vi "ModbusIRQTriggerLoop.vi"(11 "ModbusPortSettings":T1={"TxPort"="ModbusPort1Tx", "TxDataFIFO"="ModbusPort1TxFIFO", "TxInternalDataFIFO"="ModbusPort1TxInternalFIFO", "TxHealthAndStatusFIFO"="ModbusPort1TxHealthAndStatusFIFO", "RxPort"="ModbusPort1Rx", "RxDataFIFO"="ModbusPort1RxFIFO", "RxHealthAndStatusFIFO"="ModbusPort1RxHealthAndStatusFIFO", "WaitForRxFrameRegister"="ModbusPort1WaitForRxControl", "BaseHealthAndStatusAddress"=0, "IRQAddress"=0, "TriggerIRQRegister"="ModbusPort1IRQControl", "SoftwareControlledTrigger"="ModbusSoftwareControlledTrigger", "TimestampRegister"="TimestampRegister", "TxTimestampFIFO"="ModbusPort1TimestampFIFO"}) -> ()   [LabVIEW 2016, in "FPGAModbus.lvlib"]
uses:
  FPGAModbus.lvlib
  DataTypes/ModbusPortSettings.ctl
  <vilib>/rvi/Emulation/niFpgaGetClockAttributes.vi
  <vilib>/rvi/Emulation/niFpgaSctlEmulationGetInTimedLoop.vi
  <vilib>/rvi/Emulation/niFpgaEmulationReportErrorSimple.vi
  <vilib>/rvi/DataTransferAndStorage/Container/Common/niFpgaContainerExecOnDevCompGetState.vi
  <vilib>/rvi/Emulation/niFpgaEmulationIsFPGAContextNoSignature.vi
  <vilib>/rvi/DataTransferAndStorage/Container/Common/niFpgaContainerGetUniqueNameForEmu.vi
  <vilib>/rvi/Memory/Memory_Emulation/niFpgaMemoryEmulationCacheClearOnFirstRun.vi
  <vilib>/rvi/Memory/Memory_Emulation/nirvimemoryEmulationManagerCache_MakeExclusive.vi
  <vilib>/rvi/Memory/Memory_Emulation/niFpgaMemoryEmulationValidateCache.vi
  <vilib>/rvi/Memory/Memory_Emulation/nirvimemoryEmulationManagerCache_InsertValue.vi
  <vilib>/Utility/error.llb/Clear Errors.vi
  <vilib>/rvi/Memory/Memory_Emulation/nirvimemoryEmulationManagerCache_ReleaseExclusive.vi
  <vilib>/rvi/Memory/Memory_Emulation/nirvimemoryEmulationManagerCache_GetValue.vi
  <vilib>/rvi/Memory/Memory_Emulation/nirvimemoryEmulationManagerCache_SetValue.vi
  <vilib>/rvi/Emulation/niFpgaProcessEmulError.vi
  <vilib>/rvi/Emulation/niFpgaCriticalErrorInLSC.vi
  <vilib>/rvi/DataTransferAndStorage/Container/XNode/niFpgaContainer.xnode
  <vilib>/rvi/DataTransferAndStorage/Register/Emulation/niFpgaRegisterEmulationRefIn.vi
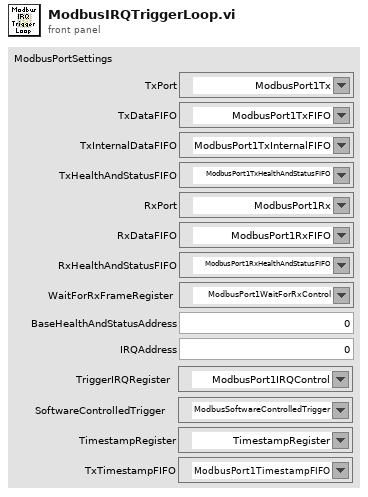
[diagram p1: front panel]
types:
  T1 = typedef "FPGAModbus.lvlib/ModbusPortSettings.ctl" = cluster{"TxPort":refnum<k21>, "TxDataFIFO":refnum<k21>, "TxInternalDataFIFO":refnum<k21>, "TxHealthAndStatusFIFO":refnum<k21>, "RxPort":refnum<k21>, "RxDataFIFO":refnum<k21>, "RxHealthAndStatusFIFO":refnum<k21>, "WaitForRxFrameRegister":refnum<k21>, "BaseHealthAndStatusAddress":u32, "IRQAddress":u8, "TriggerIRQRegister":refnum<k21>, "SoftwareControlledTrigger":refnum<k21>, "TimestampRegister":refnum<k21>, "TxTimestampFIFO":refnum<k21>}
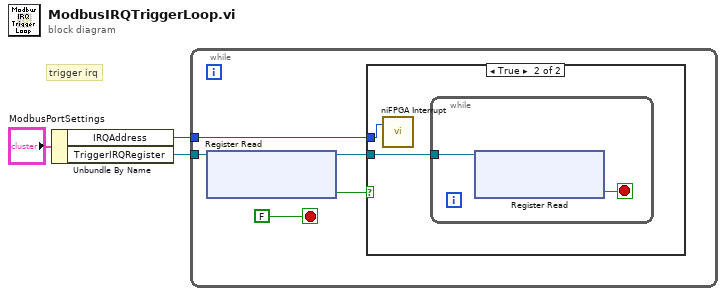
[diagram p0: block diagram]
diagram:
  # "trigger irq"
  n1 = Unbundle By Name("ModbusPortSettings") -> ("IRQAddress"=w2:u8, "TriggerIRQRegister"=w3:refnum<k21>)
  n2 = while {
    tunnel: w2 -> [w6]
    tunnel: w3 -> [w8]
    stop <- FALSE stop-if-true
    n3 = xnode ("Register Read")("Register In"=w8) -> ("Data"=w7:bool, "Register Out"=w4:refnum<k21>)
    n4 = case shown="True" w7 {
      tunnel: w6 -> [_ w10]
      tunnel: w4 -> [_ w9]
      frame False {
      }
      frame True {
        n5 = call <vilib>:"niFPGA Interrupt.vi"("IRQ Number (0)"=w10) -> ()  [unwired: 2 in]
        n6 = while {
          tunnel: w9 -> [w12]
          stop <- w11 stop-if-true
          n7 = xnode ("Register Read")("Register In"=w12) -> ("Data"=w11:bool)  [unwired: 1 out]
        }
      }
    }
  }
